vi "MQTTConfig.vi"(8 "error in (no error)":errorcluster, 10 "Jsonconfig":string, 11 "Module ID":i32) -> (0 "error out":errorcluster, 2 "Broadcasts":variant, 3 "Subscriptions":variant)   [LabVIEW 2017, in "ModbusOverMOXA.lvlib"]
uses:
  ModbusOverMOXA.lvlib
  libs/MQTT.lvlibp
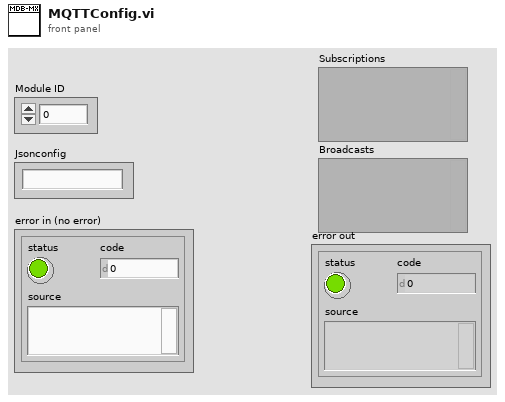
[diagram p1: front panel]
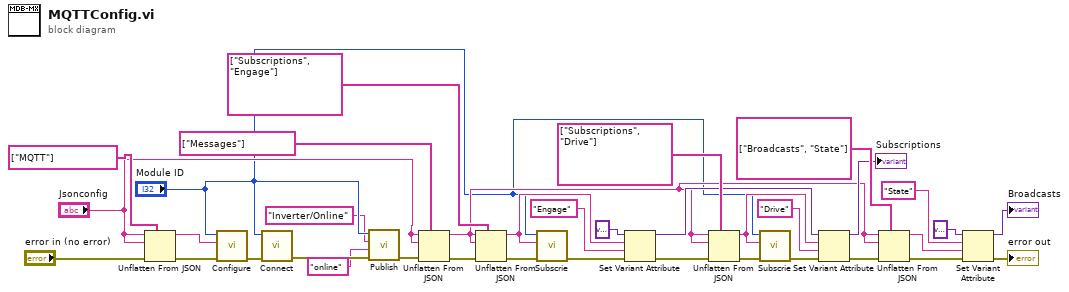
[diagram p0: block diagram]
diagram:
  n1 = Unflatten From JSON(path=string[] ["MQTT"], JSON string="Jsonconfig", type and defaults="Jsonconfig", error in (no error)="error in (no error)") -> (value=w18:string, error out=w35:errorcluster)  [unwired: 3 in]
  n2 = call "Configure.vi"("error in (no error)"=w35, "JSON config"=w18, "Module ID"="Module ID") -> ("error out"=w20:errorcluster)  [unwired: 8 in]
  n3 = call "Connect.vi"("error in (no error)"=w20, "Module ID"="Module ID") -> ("error out"=w4:errorcluster)  [unwired: 9 in]
  n4 = call "Publish.vi"("error in (no error)"=w4, "Payload"="online", "Topic"="Inverter/Online" ("name"), "Module ID"="Module ID") -> ("error out"=w5:errorcluster)  [unwired: 7 in]
  n5 = Unflatten From JSON(path=string[] ["Messages"], JSON string="Jsonconfig", type and defaults="Jsonconfig", error in (no error)=w5) -> (value=w17:string, error out=w9:errorcluster)  [unwired: 3 in]
  n6 = Unflatten From JSON(path=string[] ["Subscriptions", "Engage"], JSON string=w17, type and defaults=w17, error in (no error)=w9) -> (value=w10:string, error out=w31:errorcluster)  [unwired: 3 in]
  n7 = call "Subscrie.vi"("error in (no error)"=w31, "String"=w10, "Module ID"="Module ID") -> ("error out"=w7:errorcluster)  [unwired: 8 in]
  n8 = Set Variant Attribute(Variant=variant ("variant"), name=w10, value="Engage" ("name"), error in=w7) -> (Variant out=w27:variant, error out=w28:errorcluster)  [unwired: 1 out]
  n9 = Unflatten From JSON(path=string[] ["Subscriptions", "Drive"], JSON string=w17, type and defaults=w17, error in (no error)=w28) -> (value=w12:string, error out=w30:errorcluster)  [unwired: 3 in]
  n10 = call "Subscrie.vi"("error in (no error)"=w30, "String"=w12, "Module ID"="Module ID") -> ("error out"=w6:errorcluster)  [unwired: 8 in]
  n11 = Set Variant Attribute(Variant=w27, name=w12, value="Drive" ("name"), error in=w6) -> (Variant out=→"Subscriptions":variant, error out=w26:errorcluster)  [unwired: 1 out]
  n12 = Unflatten From JSON(path=string[] ["Broadcasts", "State"], JSON string=w17, type and defaults=w17, error in (no error)=w26) -> (value=w14:string, error out=w24:errorcluster)  [unwired: 3 in]
  n13 = Set Variant Attribute(Variant=variant ("variant"), name="State", value=w14, error in=w24) -> (Variant out=→"Broadcasts":variant, error out=→"error out":errorcluster)  [unwired: 1 out]
